vi "CAN Logfile Transfer and Convert Service (NICAN).vi"() -> ()   [LabVIEW 2010, in "CAN Log Transfer and Convert.lvlib"]
uses:
  CAN Log Transfer and Convert.lvlib
  Qd Functional Global Action.ctl
  Stop FGV Commands.ctl
  Text Format.ctl
  <vilib>/NI Veristand/Execution/Stimulus/StimulusState.ctl
  Queue Typedef.ctl
  <vilib>/NI Veristand/Execution/Stimulus/NI_VS Stimulus ExecutionAPI.lvlib
  <vilib>/ptbypt/NI_PtbyPt.lvlib
panel:
  out "Prog":u8(slide) caption="Transfer Progress" scale=0.0..100.0
  out "Queued":u16
  in  "Download":bool
  in  "NIVS.Workspace Event":refnum<event-registration>
  in  "NIVS.Project File Path":path
  in  "NIVS.Gateway IP Address":string
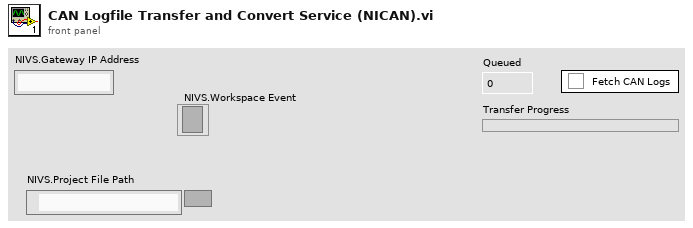
[diagram p1: front panel]
types:
  T1 = typedef "CAN Log Transfer and Convert.lvlib/Service Ref Cluster.ctl" = cluster{"queue":refnum<queue>, "Workspace":T2, "Stim":T3, "Events":cluster{"SystemChangeEventRef":T4, "NIVS.Workspace Event":refnum<event-registration>}, "SystemStateRefs":T5, "Logs folder":path, "IP":string, "CAN Sysdef":T6[]}
  T2 = typedef "NI_VS Workspace ExecutionAPI.lvlib/WorkspaceAPI.ctl" = refnum<k24>
  T3 = typedef "NI_VS Stimulus ExecutionAPI.lvlib/StimulusAPI.ctl" = refnum<k24>
  T4 = typedef "NI_VS Workspace ExecutionAPI.lvlib/SystemStateRegEventRef.ctl" = refnum<event-registration>
  T5 = typedef "NI_VS Workspace ExecutionAPI.lvlib/SystemStateEventRef.ctl" = cluster{"CustDatRef":refnum<user-event>, "EvtRef":refnum<k27>}
  T6 = typedef "CAN Log Transfer and Convert.lvlib/CAN Sysdef Data.ctl" = cluster{"Log File Name":string, "Start#":u16}
  T7 = typedef "CAN Log Transfer and Convert.lvlib/Qd Functional Global Action.ctl" = enum16{"Incr", "Reset", "Get"}
  T8 = typedef "CAN Log Transfer and Convert.lvlib/Stop FGV Commands.ctl" = enum16{"Write", "Read", "Reset"}
  T9 = typedef "NI_VS Stimulus ExecutionAPI.lvlib/StimulusState.ctl" = enum16{"Stopped", "Starting", "Running", "Stopping"}
  T10 = typedef "CAN Log Transfer and Convert.lvlib/Queue Typedef.ctl" = cluster{"Path":path, "CAN Logs":string[]}
  T11 = typedef "CAN Log Transfer and Convert.lvlib/Text Format.ctl" = enum32{"NI-CAN", "NI-XNET"}
  T12 = cluster{"SystemChangeEventRef":T4, "NIVS.Workspace Event":refnum<event-registration>}
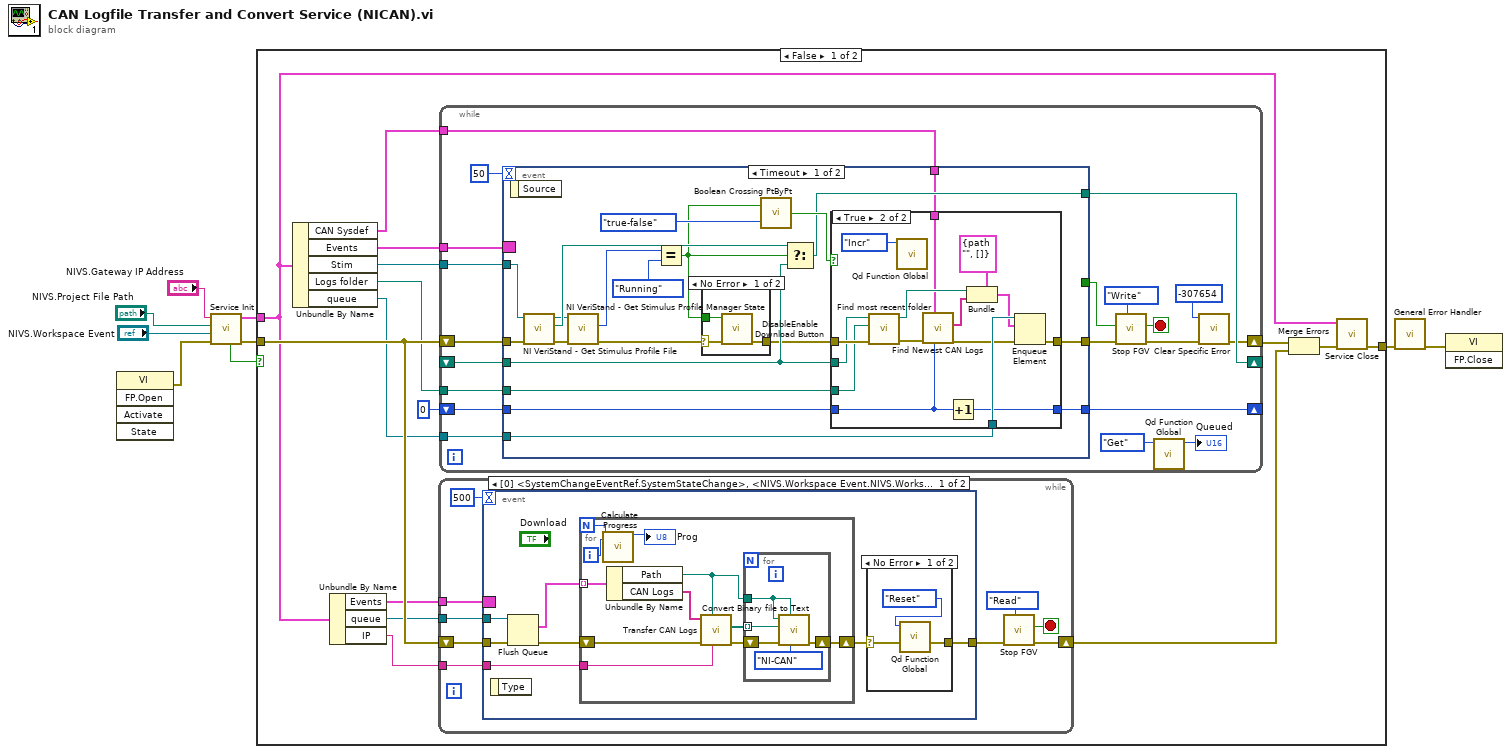
[diagram p0: block diagram]
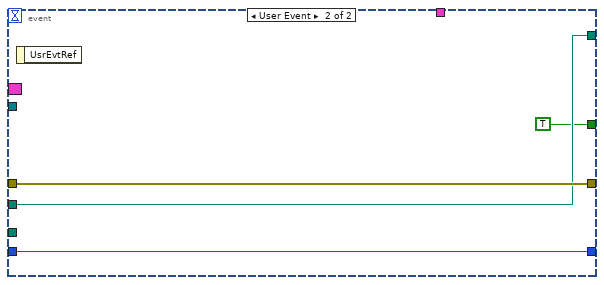
[diagram p4: hidden frame]
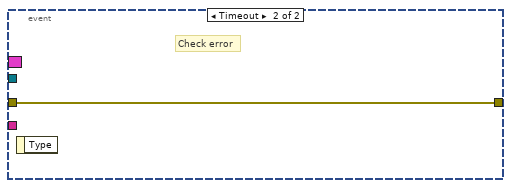
[diagram p6: hidden frame]
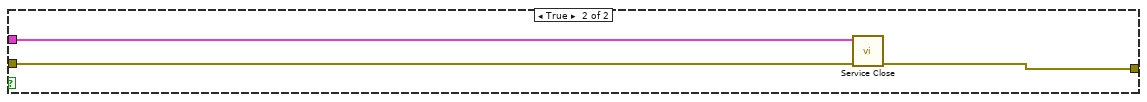
[diagram p7: hidden frame]
diagram:
  n1 = invoke class="VI" method="FP.Open"() -> (error out=w2:errorcluster)  [unwired: 5 in, 4 out]
  n2 = call "Service Init.vi"("error in (no error)"=w2, "NIVS.Workspace Event"="NIVS.Workspace Event", "NIVS.Project File Path"="NIVS.Project File Path", "NIVS.Gateway IP Address"="NIVS.Gateway IP Address") -> ("error out"=w7:errorcluster, "System Refs Cluster"=w6:T1, "No CAN Logs"=w5:bool)  [unwired: 5 in]
  n3 = case shown="False" w5 {
    tunnel: w7 -> [w24 w127]
    tunnel: [w10 w128] -> w4
    tunnel: w6 -> [w16 w126]
    frame False {
      n4 = Unbundle By Name(w16) -> ("CAN Sysdef"=w18:T6[], "Events"=w17:T12, "Stim"=w23:T3, "Logs folder"=w22:path, "queue"=w21:refnum<queue>)
      n5 = Unbundle By Name(w16) -> ("Events"=w14:T12, "queue"=w20:refnum<queue>, "IP"=w19:string)
      n6 = while {
        shift-right: [w97] -> w15
        shift-left: w24 -> [w98]
        tunnel: w20 -> [w95]
        tunnel: w19 -> [w94]
        tunnel: w14 -> [w91]
        stop <- w93 stop-if-true
        n7 = event shown="[0] <SystemChangeEventRef.SystemStateChange>, <NIVS.Workspace Event.NIVS.Workspace Event>: User Event;  \"Download\": Value Change" {
          selector: w91 -> [_ _]
          dyn-events: _ -> [_ _]
          timeout: 500 -> [_ _]
          tunnel: w98 -> [w105 w125]
          tunnel: w95 -> [w104 _]
          tunnel: w94 -> [w102 _]
          tunnel: [w99 w125] -> w92
          event User Event; "Download": Value Change {
            n8 = event-data() -> ()  [unwired: 1 in, 1 out]
            n9 = Flush Queue(queue=w104, error in (no error)=w105) -> (remaining elements=w101:T10[], error out=w103:errorcluster)  [unwired: 1 out]
            n10 = for {
              N -> [w110]
              tunnel: w102 -> [w117]
              tunnel: w101 -> [w112] mode=indexing
              shift-right: [w119] -> w100
              shift-left: w103 -> [w118]
              i -> [w111]
              n11 = call "Calculate Progress.vi"("Total Iterations"=w110, "Current Iteration"=w111) -> ("Progress"=→"Prog":u8)  [unwired: 17 in]
              n12 = Unbundle By Name(w112) -> ("Path"=w115:path, "CAN Logs"=w114:string[])
              n13 = call "Transfer CAN Logs.vi"("address"=w117, "Destination"=w115, "error in (no error)"=w118, "Raw CAN Log files"=w114) -> ("error out"=w116:errorcluster, "Files moved"=w113:path[])  [unwired: 6 in]
              n14 = for {
                shift-right: [w122] -> w119
                shift-left: w116 -> [w123]
                tunnel: w115 -> [w121]
                tunnel: w113 -> [w120] mode=indexing
                n15 = call "Convert Binary file to Text.vi"("Text format"=Text_Format."NI-CAN", "Originating directory"=w121, "error in (no error)"=w123, "NCL File Path"=w120, "Destination directory"=w121) -> ("error out"=w122:errorcluster)  [unwired: 6 in]
              }
            }
            n16 = case shown="No Error" w100 {
              selector: w100 -> [w107 w108]
              tunnel: [w107 w108] -> w99
              frame No Error {
                n17 = call "Qd Function Global.vi"("Action"=Qd_Functional_Global_Action."Reset") -> ()  [unwired: 10 in, 1 out]
              }
              frame Error {
              }
            }
          }
          event Timeout {
            # "Check error"
            n18 = event-data() -> ()  [unwired: 1 in, 1 out]
          }
        }
        n19 = call "Stop FGV.vi"("Command"=Stop_FGV_Commands."Read", "error in (no error)"=w92) -> ("error out"=w97:errorcluster, "Latched Stop"=w93:bool)  [unwired: 7 in, 1 out]
      }
      n20 = while {
        shift-right: [w42] -> _
        shift-left: _ -> [w41]
        shift-right: [w29] -> w12
        shift-left: w24 -> [w44]
        tunnel: w23 -> [w38]
        tunnel: w22 -> [w37]
        tunnel: w21 -> [w36]
        tunnel: w18 -> [w35]
        tunnel: w17 -> [w34]
        shift-right: [w27] -> _
        shift-left: u16 0 -> [w28]
        stop <- w33 stop-if-true
        n21 = event shown="[0] Timeout" {
          selector: w34 -> [_ _]
          dyn-events: _ -> [_ _]
          timeout: 50 -> [_ _]
          tunnel: [w50 w89] -> w32
          tunnel: w44 -> [w57 w89]
          tunnel: [_ TRUE] -> w39
          tunnel: [w60 w88] -> w42
          tunnel: w41 -> [w59 w88]
          tunnel: w38 -> [w54 _]
          tunnel: w37 -> [w53 _]
          tunnel: w36 -> [w52 _]
          tunnel: w35 -> [w51 _]
          tunnel: w28 -> [w49 w86]
          tunnel: [w48 w86] -> w27
          event Timeout {
            n22 = event-data() -> ()  [unwired: 1 in, 1 out]
            n23 = call <vilib>:"NI VeriStand - Get Stimulus Profile File.vi"("error in (no error)"=w57, "StimulusProfileManager in"=w54) -> ("error out"=w56:errorcluster, "File"=w58:path, "StimulusProfileManager out"=w55:T3)  [unwired: 7 in]
            n24 = call <vilib>:"NI VeriStand - Get Stimulus Profile Manager State.vi"("error in (no error)"=w56, "StimulusProfileManager in"=w55) -> ("error out"=w46:errorcluster, "State"=w64:T9)  [unwired: 7 in, 1 out]
            n25 = Equal?(x=w64, y=StimulusState."Running") -> (x = y?=w45:bool)
            n26 = case shown="No Error" w46 {
              selector: w46 -> [w67 w68]
              tunnel: [w66 w68] -> w47
              tunnel: w45 -> [w65 _]
              frame No Error {
                n27 = call "DisableEnable Download Button.vi"("error in (no error)"=w67, "Disable?"=w65) -> ("error out"=w66:errorcluster)  [unwired: 9 in]
              }
              frame Error {
              }
            }
            n28 = call <vilib>:"Boolean Crossing PtByPt.vi"("direction"=enum16{"either", "false-true", "true-false"}."true-false", "input"=w45) -> ("crossing"=w61:bool)  [unwired: 1 in]
            n29 = Select(t=w58, s=w45, f=w59) -> (s? t:f=w60:path)
            n30 = case shown="True" w61 {
              tunnel: w47 -> [w70 w85]
              tunnel: [w70 w83] -> w50
              tunnel: w59 -> [_ w82]
              tunnel: w53 -> [_ w81]
              tunnel: w52 -> [_ w84]
              tunnel: w51 -> [_ w74]
              tunnel: w49 -> [w69 w73]
              tunnel: [w69 w72] -> w48
              frame False {
              }
              frame True {
                n31 = call "Find most recent folder.vi"("error in (no error)"=w85, "Directory to search"=w81, "File path (used for pattern search)"=w82) -> ("error out"=w80:errorcluster, "most recent folder"=w78:path)  [unwired: 7 in]
                n32 = call "Qd Function Global.vi"("Action"=Qd_Functional_Global_Action."Incr") -> ()  [unwired: 10 in, 1 out]
                n33 = call "Find Newest CAN Logs.vi"("# Queued"=w73, "CAN Sysdef Config"=w74, "error in (no error)"=w80) -> ("error out"=w75:errorcluster, "Files To Transfer"=w77:string[])  [unwired: 7 in]
                n34 = Increment(x=w73) -> (x+1=w72:u16)
                n35 = Bundle(cluster=T10 {"Path"=path "", "CAN Logs"=[]} ("Queue Data"), "Path"=w78, "CAN Logs"=w77) -> (w76:T10)
                n36 = Enqueue Element(queue=w84, element=w76, error in (no error)=w75) -> (error out=w83:errorcluster)  [unwired: 1 in, 2 out]
              }
            }
          }
          event User Event {
            n37 = event-data() -> ()  [unwired: 1 in, 1 out]
          }
        }
        n38 = call "Stop FGV.vi"("Command"=Stop_FGV_Commands."Write", "error in (no error)"=w32, "Stop?"=w39) -> ("error out"=w30:errorcluster, "Latched Stop"=w33:bool)  [unwired: 6 in, 1 out]
        n39 = call "Qd Function Global.vi"("Action"=Qd_Functional_Global_Action."Get") -> ("Queued"=→"Queued":u16)  [unwired: 10 in]
        n40 = call "Clear Specific Error.vi"("error in (no error)"=w30, "code"=-307654 ("y")) -> ("error out"=w29:errorcluster)  [unwired: 9 in]
      }
      n41 = Merge Errors(w12, w15) -> (w11:errorcluster)
      n42 = call "Service Close.vi"("error in (no error)"=w11, "Service Refs Cluster"=w16) -> ("error out"=w10:errorcluster)  [unwired: 9 in]
    }
    frame True {
      n43 = call "Service Close.vi"("error in (no error)"=w127, "Service Refs Cluster"=w126) -> ("error out"=w128:errorcluster)  [unwired: 9 in]
    }
  }
  n44 = call <vilib>:"General Error Handler.vi"("error in (no error)"=w4) -> ("error out"=w1:errorcluster)  [unwired: 10 in, 4 out]
  n45 = invoke class="VI" method="FP.Close"(error in=w1) -> ()  [unwired: 2 in, 3 out]
